vi "ReadAIs.vi"(8 "error in (no error)":errorcluster, 10 "Analog Inputs":T1, 11 "VISA resource name":refnum<visa-resource-name>) -> (0 "error out":errorcluster, 2 "Value":u16, 3 "VISA resource name out":refnum<visa-resource-name>)   [LabVIEW 2023, in "HandsOnPi2040.lvlib"]
uses:
  <instrlib>/HandsOnPi2040/HandsOnPi2040.lvlib
  <instrlib>/HandsOnPi2040/Public/AnaIns.ctl
  <instrlib>/HandsOnPi2040/cti-drivers-lv-visa-main/CTI-Visa/CTI-Visa.lvlib
panel:
  # "Output"
  # "Input"
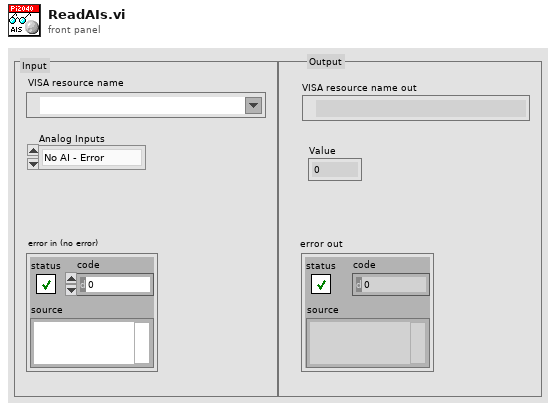
[diagram p1: front panel]
types:
  T1 = typedef "HandsOnPi2040.lvlib/AnaIns.ctl" = enum16{"No AI - Error", "AI1 (GPIO26)", "AI2 (GPIO27)"}
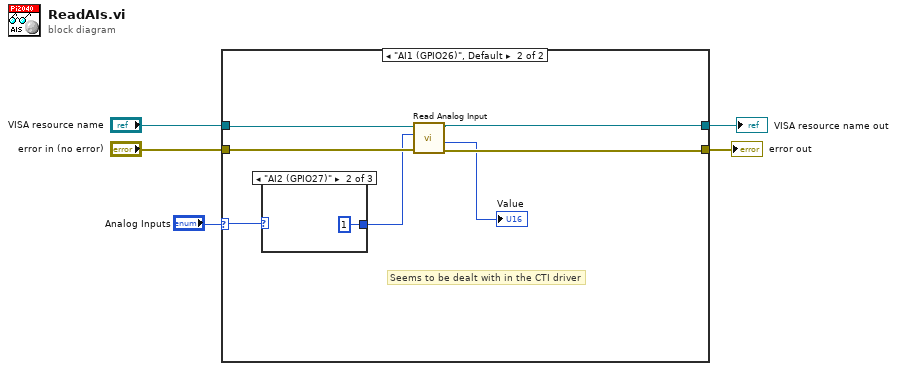
[diagram p0: block diagram]
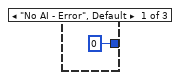
[diagram p3: hidden frame]
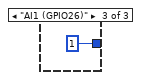
[diagram p4: hidden frame]
diagram:
  n1 = case shown="\"AI1 (GPIO26)\", Default" "Analog Inputs" {
    selector: "Analog Inputs" -> [_ w9]
    tunnel: "VISA resource name" -> [w6 w14]
    tunnel: "error in (no error)" -> [w7 w13]
    tunnel: [w6 w11] -> w5
    tunnel: [w7 w12] -> w4
    frame "No AI - Error" {
    }
    frame "AI1 (GPIO26)", Default {
      # "Seems to be dealt with in the CTI driver"
      n2 = case shown="\"AI2 (GPIO27)\"" w9 {
        tunnel: [0 ("Channel") 1 ("Channel") 1 ("Channel")] -> w8
        frame "No AI - Error", Default {
        }
        frame "AI2 (GPIO27)" {
        }
        frame "AI1 (GPIO26)" {
        }
      }
      n3 = call <instrlib>:"Read Analog Input.vi"("error in (no error)"=w13, "Channel"=w8, "VISA resource name in"=w14) -> ("error out"=w12:errorcluster, "Value"=→"Value":u16, "VISA resource name"=w11:refnum<visa-resource-name>)  [unwired: 6 in]
    }
  }
  "VISA resource name out" <- w5
  "error out" <- w4
